vi "Stop Core.vi"(10 "final error code":i32, 11 "Output Actor Hardware in":refnum<class "Output Actor Hardware.lvclass">) -> (3 "Output Actor Hardware out":refnum<class "Output Actor Hardware.lvclass">)   [LabVIEW 2015, in "Output Actor Hardware.lvclass"]
doc: "(<B>Filename</B>: Actor Framework.lvlib:Actor.lvclass:Stop Core.vi)\n\nDefines what the actor does before it stops. Use the <B>final error code</B> input to determine whether the actor shut down in response to an error.\n\nBy default, this method does nothing. A descendant class may override it to define behavior, such as shutting down any processes the actor initiated in its override of the Actor Core method."
uses:
  Output Actor Hardware.lvclass
  Output Actor Hardware.lvclass/Output Actor Hardware.ctl
  output actor/Output Actor.lvclass
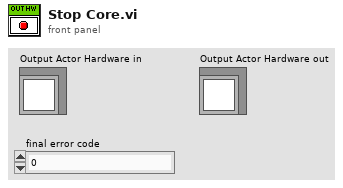
[diagram p1: front panel]
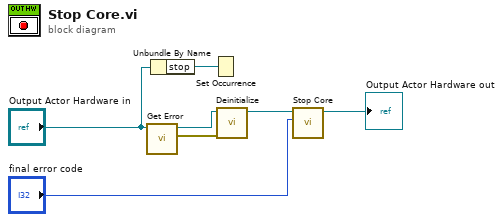
[diagram p0: block diagram]
diagram:
  n1 = call "Get Error.vi"("Output Actor Hardware in"="Output Actor Hardware in") -> ("Error"=w4:errorcluster, "Output Actor Hardware out"=w3:refnum<class "Output Actor Hardware.lvclass">)  [unwired: 8 in, 1 out]
  n2 = Unbundle By Name("Output Actor Hardware in") -> ("stop"=w5:refnum<k4>)
  n3 = Set Occurrence(w5) -> ()
  n4 = call-dynamic "Deinitialize.vi"("error in (no error)"=w4, "Output Actor Hardware in"=w3) -> ("Output Actor Hardware out"=w1:refnum<class "Output Actor Hardware.lvclass">)  [unwired: 9 in]
  n5 = call-parent "Stop Core.vi"("final error code"="final error code", "Actor in"=w1) -> ("Actor out"=→"Output Actor Hardware out":refnum<class "Output Actor Hardware.lvclass">)  [unwired: 9 in]
